vi "Read Waveform Measurement (Px Statistics).vi"(0 "VISA resource name":refnum<visa-resource-name>, 5 "Parameter (0: P1)":u16(ring) items=["P1", "P2", "P3", "P4", "P5", "P6", "P7", "P8", "P9", "P10", "P11", "P12"], 11 "error in (no error)":errorcluster) -> (2 "Min":dbl format="%#_6e", 3 "Max":dbl format="%#_6e", 4 "VISA resource name out":refnum<visa-resource-name>, 6 "Value":dbl format="%#_6e", 8 "Sigma":dbl format="%#_6e", 10 "num":dbl format="%#_6f", 12 "StatusDescription":string, 13 "Mean":dbl format="%#_6e", 14 "enabled?":bool, 15 "error out":errorcluster)   [LabVIEW 2018, in "LeCroy Wave Series.lvlib"]
doc: "This VI reads back all statistics for a parameter previously configured on P1 - P8. P1-P5 are available on most scopes; availability is model dependant.\n\n(The statistics table does not need to be visible on the scope to use this VI)"
uses:
  LeCroy Wave Series.lvlib
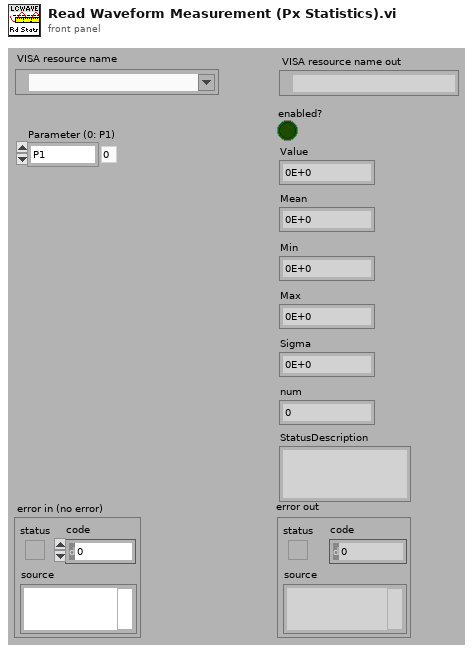
[diagram p1: front panel]
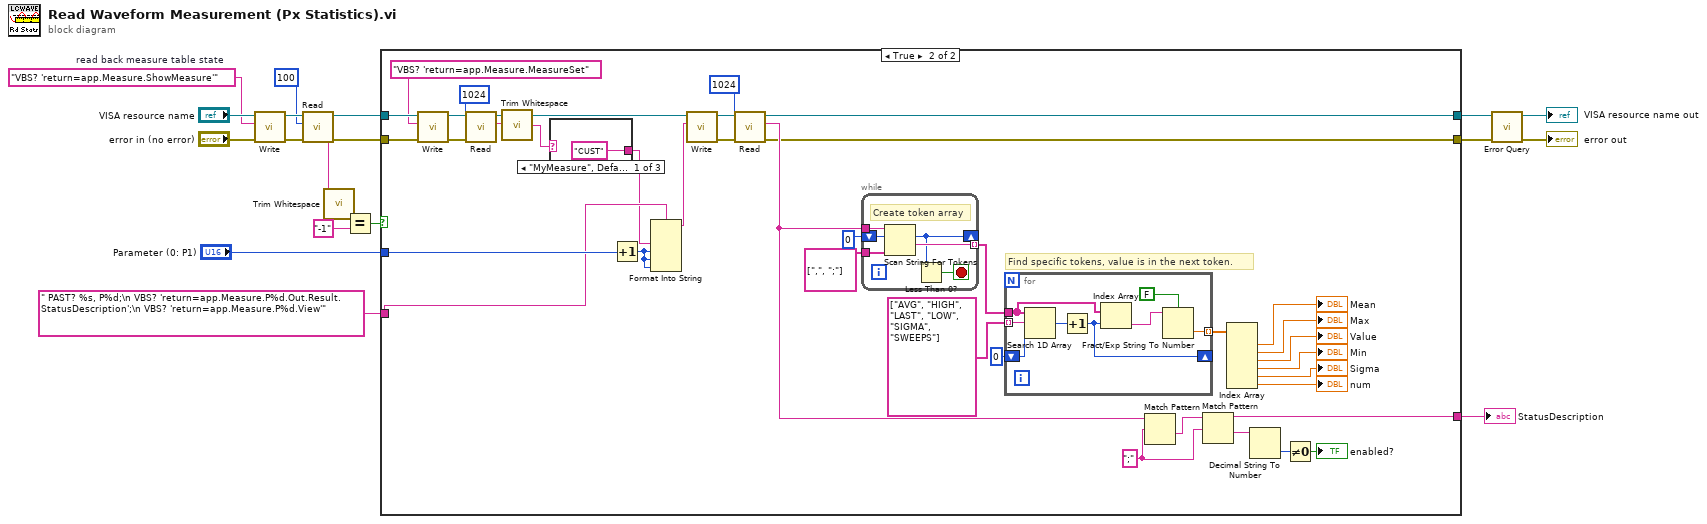
[diagram p0: block diagram]
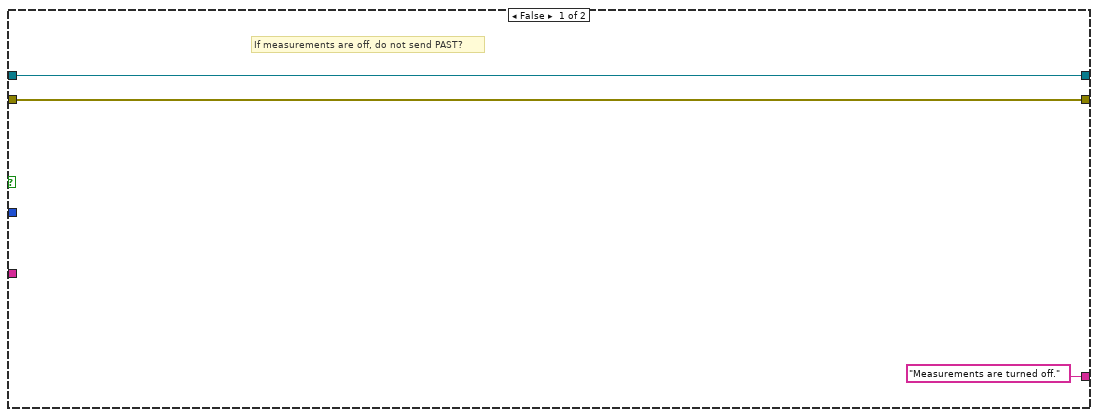
[diagram p2: hidden frame]
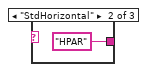
[diagram p3: hidden frame]
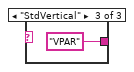
[diagram p4: hidden frame]
diagram:
  w15 = "VBS? 'return=app.Measure.ShowMeasure'"  # read back measure table state
  n1 = call "Write.vi"("error in (no error)"="error in (no error)", "Write Buffer"=w15, "VISA resource name"="VISA resource name") -> ("error out"=w14:errorcluster, "VISA resource name out"=w18:refnum<visa-resource-name>)  [unwired: 7 in]
  n2 = call "Read.vi"("error in (no error)"=w14, "Byte Count"=u32 100, "VISA resource name"=w18) -> ("error out"=w10:errorcluster, "Read Buffer"=w2:string, "VISA resource name out"=w12:refnum<visa-resource-name>)  [unwired: 5 in, 1 out]
  n3 = call <vilib>:"Trim Whitespace.vi"("string"=w2) -> ("trimmed string"=w1:string)  [unwired: 1 in]
  n4 = Equal?(x=w1, y="-1") -> (x = y?=w4:bool)
  n5 = case shown="True" w4 {
    tunnel: ["Measurements are turned off." ("Read Buffer") w38] -> w19
    tunnel: w12 -> [w20 w30]
    tunnel: "Parameter (0: P1)" -> [_ w36]
    tunnel: w10 -> [w21 w29]
    tunnel: [w21 w35] -> w7
    tunnel: [w20 w34] -> w6
    tunnel: " PAST? %s, P%d;\n VBS? 'return=app.Measure.P%d.Out.Result.StatusDescription';\n VBS? 'return=app.Measure.P%d.View'" ("format string") -> [_ w33]
    frame False {
      # "If measurements are off, do not send PAST?"
    }
    frame True {
      w42 = ";" ("regular expression")
      # "Find specific tokens, value is in the next token."
      n6 = call "Write.vi"("error in (no error)"=w29, "Write Buffer"="VBS? 'return=app.Measure.MeasureSet" ("read back measure table state"), "VISA resource name"=w30) -> ("error out"=w28:errorcluster, "VISA resource name out"=w32:refnum<visa-resource-name>)  [unwired: 7 in]
      n7 = call "Read.vi"("error in (no error)"=w28, "Byte Count"=u32 1024, "VISA resource name"=w32) -> ("Read Buffer"=w25:string, "VISA resource name out"=w26:refnum<visa-resource-name>)  [unwired: 5 in, 2 out]
      n8 = call <vilib>:"Trim Whitespace.vi"("string"=w25) -> ("trimmed string"=w24:string)  [unwired: 1 in]
      n9 = case shown="\"MyMeasure\", Default" w24 {
        tunnel: ["CUST" "HPAR" "VPAR"] -> w23
        frame "MyMeasure", Default {
        }
        frame "StdHorizontal" {
        }
        frame "StdVertical" {
        }
      }
      n10 = Increment(x=w36) -> (x+1=w37:u16)
      n11 = Format Into String(format string=w33, w23, w37, w37, w37) -> (resulting string=w58:string)  [unwired: 2 in, 1 out]
      n12 = call "Write.vi"("Write Buffer"=w58, "VISA resource name"=w26) -> ("error out"=w59:errorcluster, "VISA resource name out"=w60:refnum<visa-resource-name>)  [unwired: 8 in]
      n13 = call "Read.vi"("error in (no error)"=w59, "Byte Count"=u32 1024, "VISA resource name"=w60) -> ("error out"=w35:errorcluster, "Read Buffer"=w44:string, "VISA resource name out"=w34:refnum<visa-resource-name>)  [unwired: 5 in, 1 out]
      n14 = while {
        tunnel: w44 -> [w77]
        tunnel: string[] [",", ";"] ("delimiters (\\s,\\t,\\r,\\n)") -> [w76]
        shift-right: [w72] -> _
        shift-left: 0 ("offset past token") -> [w75]
        tunnel: [w74] -> w53 mode=indexing
        stop <- w73 stop-if-true
        # "Create token array"
        n15 = Scan String For Tokens(6:w76, 8:w75, 9:w77) -> (1:w74:string, 2:w72:i32)  [unwired: 3 in, 2 out]
        n16 = Less Than 0?(x=w72) -> (x < 0?=w73:bool)
      }
      n17 = for {
        tunnel: w53 -> [w67]
        tunnel: string[] ["AVG", "HIGH", "LAST", "LOW", "SIGMA", "SWEEPS"] -> [w71] mode=indexing
        shift-right: [w68] -> _
        shift-left: 0 -> [w69]
        tunnel: [w64] -> w51 mode=indexing
        n18 = Search 1D Array(1D array=w67, element=w71, start index (0)=w69) -> (index of element=w70:i32)
        n19 = Increment(x=w70) -> (x+1=w68:i32)
        n20 = Index Array(array=w67, index=w68) -> (element=w66:string)
        n21 = Fract/Exp String To Number(use system decimal point (T)=FALSE, string=w66) -> (number=w64:dbl)  [unwired: 2 in, 1 out]
      }
      n22 = Match Pattern(string=w44, regular expression=w42) -> (after substring=w43:string)  [unwired: 1 in, 3 out]
      n23 = Match Pattern(string=w43, regular expression=w42) -> (before substring=w38:string, after substring=w41:string)  [unwired: 1 in, 2 out]
      n24 = Index Array(array=w51) -> (element #1=→"Mean":dbl, element #2=→"Max":dbl, element #3=→"Value":dbl, element #4=→"Min":dbl, element #5=→"Sigma":dbl, element #6=→"num":dbl)  [unwired: 6 in]
      n25 = Decimal String To Number(string=w41) -> (number=w40:i32)  [unwired: 2 in, 1 out]
      n26 = Not Equal To 0?(x=w40) -> (x != 0?=→"enabled?":bool)
    }
  }
  "StatusDescription" <- w19
  n27 = call "Error Query.vi"("error in (no error)"=w7, "VISA resource name"=w6) -> ("error out"=→"error out":errorcluster, "VISA resource name out"=→"VISA resource name out":refnum<visa-resource-name>)  [unwired: 6 in, 2 out]
